vi "RTS Get StartStop Time Door Ops.vi"(8 "Error In":errorcluster, 11 "Door Op Data Input":string[][](array[string])) -> (0 "Error Out":errorcluster, 1 "End Time":timestamp, 2 "Start Time":timestamp, 3 "Door Op Data Output":string[][](array[string]), 5 "Elapsed days":i32)   [LabVIEW 2016]
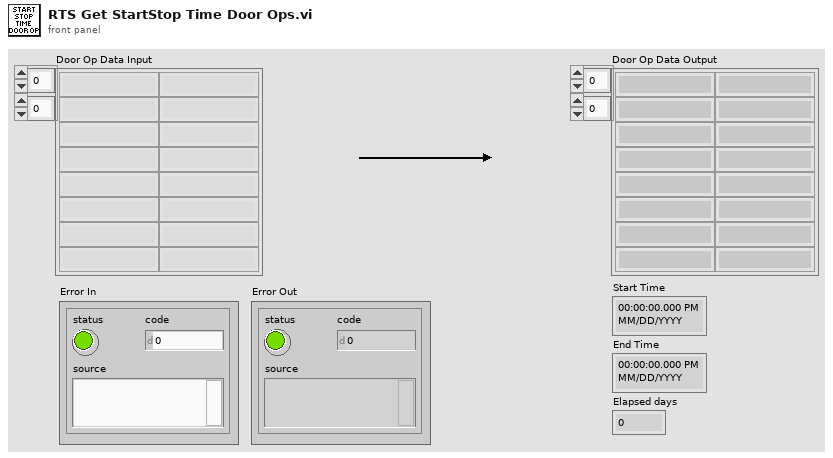
[diagram p1: front panel]
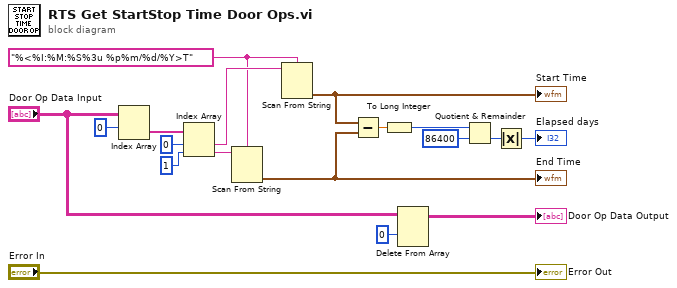
[diagram p0: block diagram]
diagram:
  w10 = "%<%I:%M:%S%3u %p%m/%d/%Y>T" ("format string")
  n1 = Index Array(array="Door Op Data Input", index (row)=0) -> (element=w15:string[])  [unwired: 1 in]
  n2 = Index Array(array=w15, index #1=0 ("index"), index #2=1 ("index")) -> (element #1=w12:string, element #2=w11:string)
  n3 = Scan From String(format string=w10, input string=w11) -> (output 1=w18:timestamp)  [unwired: 3 in, 3 out]
  "End Time" <- w18
  n4 = Scan From String(format string=w10, input string=w12) -> (output 1=w17:timestamp)  [unwired: 3 in, 3 out]
  "Start Time" <- w17
  n5 = Subtract(x=w17, y=w18) -> (x-y=w7:dbl)
  n6 = To Long Integer(number=w7) -> (32bit integer=w9:i32)
  n7 = Delete From Array(array="Door Op Data Input", index (row)=0) -> (array with subset deleted=→"Door Op Data Output":string[][])  [unwired: 2 in, 1 out]
  n8 = Quotient & Remainder(x=w9, y=86400) -> (floor(x/y)=w6:i32)  [unwired: 1 out]
  n9 = Absolute Value(x=w6) -> (abs(x)=→"Elapsed days":i32)
  "Error Out" <- "Error In"
